vi "LEB Decoder.vi"(11 "encoded string":string) -> (0 "bytes consumed":i32, 2 "unmodified string":string, 3 "Number":u32)   [LabVIEW 2017]
doc: "Decode the first few bytes assuming LEB128 encoding. This is how Java and C++ NT clients chose to implement their lengths for strings and arrays."
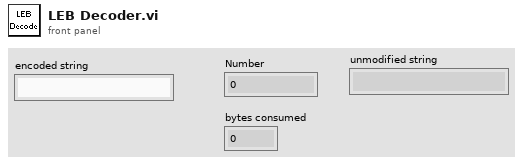
[diagram p1: front panel]
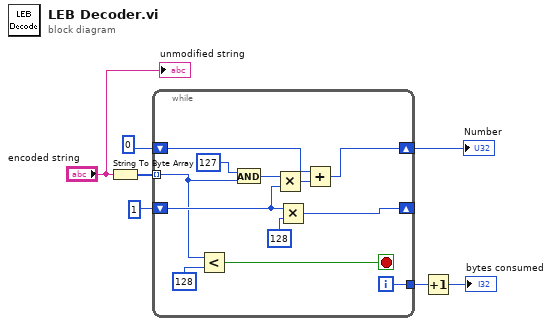
[diagram p0: block diagram]
diagram:
  n1 = String To Byte Array(string="encoded string") -> (unsigned byte array=w7:u8[])
  n2 = while {
    tunnel: w7 -> [w10] mode=indexing
    shift-right: [w18] -> w5
    shift-left: u32 0 -> [w19]
    shift-right: [w16] -> _
    shift-left: u32 1 -> [w17]
    tunnel: [w8] -> w3
    i -> [w8]
    stop <- w12 stop-if-true
    n3 = Less?(x=w10, y=u32 128) -> (x < y?=w12:bool)
    n4 = And(x=u8 127, y=w10) -> (x .and. y?=w11:u8)
    n5 = Multiply(x=w11, y=w17) -> (x*y=w14:u32)
    n6 = Multiply(x=w17, y=u32 128) -> (x*y=w16:u32)
    n7 = Add(x=w19, y=w14) -> (x+y=w18:u32)
  }
  "Number" <- w5
  n8 = Increment(x=w3) -> (x+1=→"bytes consumed":i32)
  "unmodified string" <- "encoded string"
